vi "USBSelfTest.vi"(9 "error in (no error)":errorcluster) -> (1 "error out":errorcluster, 2 "USB":string, 4 "CmdOut":string)   [LabVIEW 2013]
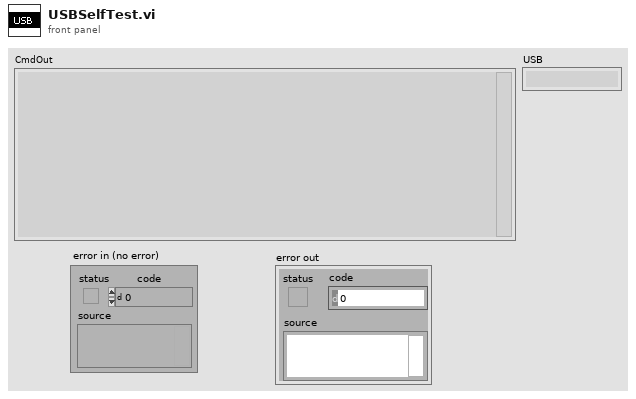
[diagram p1: front panel]
types:
  T1 = enum32{"invalid app kind", "Development System", "Run Time System", "Student Edition", "Embedded LabVIEW", "Evaluation", "Custom"}
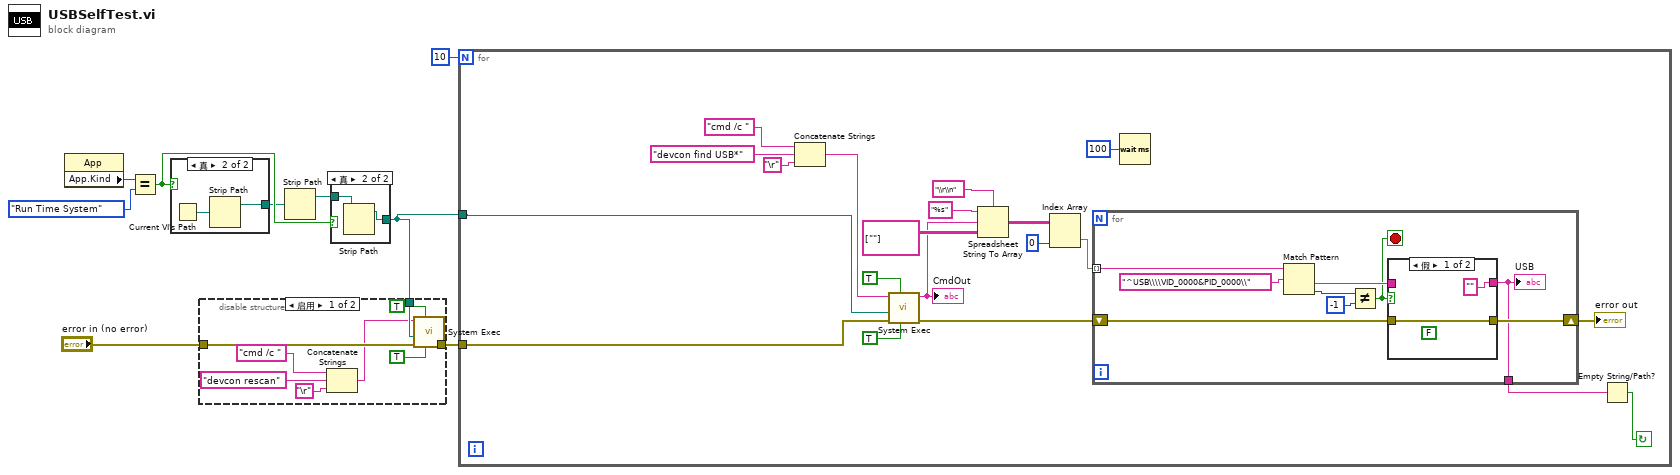
[diagram p0: block diagram]
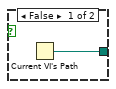
[diagram p4: hidden frame]
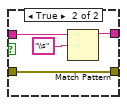
[diagram p5: hidden frame]
diagram:
  n1 = property class="App"() -> ("App.Kind"=w5:T1)  [unwired: 2 in, 2 out]
  n2 = Equal?(x=w5, y=T1."Run Time System") -> (x = y?=w7:bool)
  n3 = case shown="真" w7 {
    tunnel: [w10 w12] -> w6
    frame False {
      n4 = Current VI's Path() -> (path=w10:path)
    }
    frame True {
      n5 = Current VI's Path() -> (path=w11:path)
      n6 = Strip Path(path=w11) -> (stripped path=w12:path)  [unwired: 1 out]
    }
  }
  n7 = Strip Path(path=w6) -> (stripped path=w8:path)  [unwired: 1 out]
  n8 = case shown="真" w7 {
    tunnel: w8 -> [w13 w15]
    tunnel: [w13 w14] -> w1
    frame False {
    }
    frame True {
      n9 = Strip Path(path=w15) -> (stripped path=w14:path)  [unwired: 1 out]
    }
  }
  n10 = disable-structure shown="启用" {
    disable-tunnel: [w24 w25] -> w2
    disable-tunnel: "error in (no error)" -> [w23 w25]
    disable-tunnel: w1 -> [w22 _]
    frame Enabled {
      n11 = Concatenate Strings("cmd /c " ("command line"), "devcon rescan" ("command"), "\r") -> (w18:string)
      n12 = call <vilib>:"System Exec.vi"("run minimized? (F)"=TRUE, "wait until completion? (T)"=TRUE, "error in (no error)"=w23, "working directory"=w22, "command line"=w18) -> ("error out"=w24:errorcluster)  [unwired: 1 in, 5 out]
    }
    frame Disabled {
    }
  }
  n13 = for {
    N: 10 -> [_]
    tunnel: w1 -> [w27]
    tunnel: w2 -> [w26]
    stop <- w28 continue-if-true
    n14 = Concatenate Strings("cmd /c " ("command line"), "devcon find USB*" ("command"), "\r") -> (w43:string)
    n15 = call <vilib>:"System Exec.vi"("run minimized? (F)"=TRUE, "wait until completion? (T)"=TRUE, "error in (no error)"=w26, "working directory"=w27, "command line"=w43) -> ("error out"=w32:errorcluster, "standard output"=w34:string)  [unwired: 1 in, 4 out]
    "CmdOut" <- w34
    n16 = Spreadsheet String To Array(delimiter (Tab)="\\r\\n" ("格式字符串"), format string="%s" ("格式字符串"), spreadsheet string=w34, array type (2D Dbl)=string[][] [[""]]) -> (array=w36:string[][])
    n17 = Index Array(array=w36, index (col)=0 ("索引 (行)")) -> (element=w33:string[])  [unwired: 1 in]
    n18 = for {
      tunnel: w33 -> [w50] mode=indexing
      shift-right: [w48] -> w31
      shift-left: w32 -> [w49]
      tunnel: [w46] -> w29
      stop <- w47 stop-if-true
      n19 = Match Pattern(string=w50, regular expression="^USB\\\\VID_0000&PID_0000\\" ("command line")) -> (after substring=w54:string, offset past match=w52:i32)  [unwired: 3 out]
      n20 = Not Equal?(x=w52, y=-1) -> (x != y?=w47:bool)
      n21 = case shown="假" w47 {
        tunnel: w54 -> [_ w59]
        tunnel: w49 -> [w56 w57]
        tunnel: [w56 w57] -> w48
        tunnel: ["" w58] -> w46
        frame False {
          (unwired) FALSE
        }
        frame True {
          n22 = Match Pattern(string=w59, regular expression="\\s" ("正则表达式")) -> (before substring=w58:string)  [unwired: 4 out]
        }
      }
      "USB" <- w46
    }
    "error out" <- w31
    n23 = Wait (ms)(milliseconds to wait=u32 100 ("等待时间（毫秒）")) -> ()  [unwired: 1 out]
    n24 = Empty String/Path?(string/path=w29) -> (empty?=w28:bool)
  }
